vi "svfa_Check Waveform Parameter Continuity (1x1) [Dual FFT].vi"(0 "stimulus signal X [EUx]":waveform(dbl), 1 "restart averaging (F)":bool, 5 "response signal Y [EUy]":waveform(dbl), 7 "checks for channel parameter change":T1={"dt"=TRUE, "t0 continuity"=FALSE, "array length"=TRUE, "channel info"=TRUE, "name"=FALSE}, 11 "error in":errorcluster) -> (3 "dt":dbl, 4 "stimulus signal X [EUx]":waveform(dbl), 6 "response signal Y [EUy]":waveform(dbl), 8 "waveform parameter changed":bool, 14 "array length":i32, 15 "error out":errorcluster)   [LabVIEW 2017]
uses:
  <vilib>/addons/_NISVFA/_Shared subVIs/Common/svc_Check for Waveform Parameter Continuity (no state).vi
  <vilib>/addons/_NISVFA/_Shared subVIs/Common/svc_Get SV Channel Info.vi
  <vilib>/addons/_NISVFA/_Shared subVIs/Common/svc_Engineering Units to Unit Label.vi
  <vilib>/addons/_NISVFA/_Shared subVIs/Common/svc_Unit Label to Engineering Units.vi
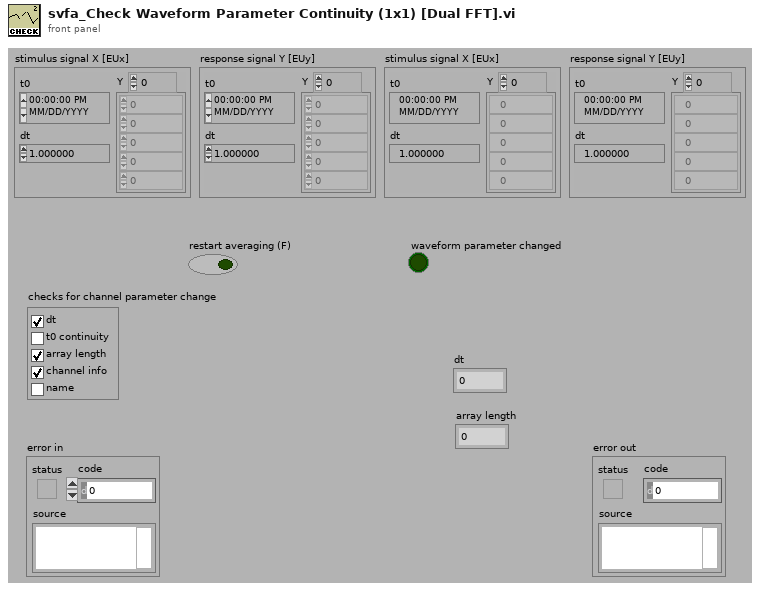
[diagram p1: front panel]
types:
  T1 = cluster{"dt":bool, "t0 continuity":bool, "array length":bool, "channel info":bool, "name":bool}
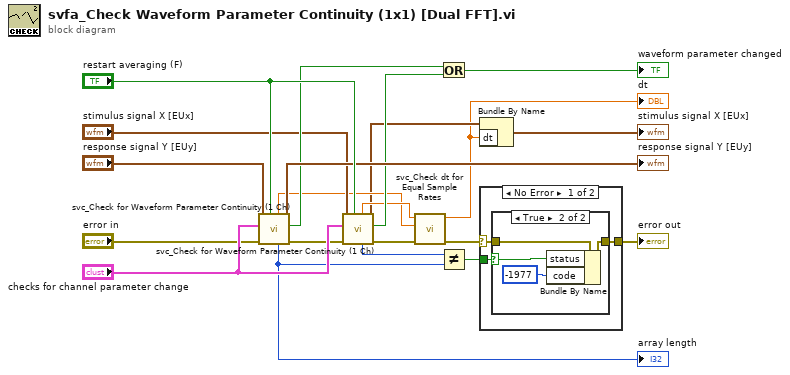
[diagram p0: block diagram]
diagram:
  n1 = call <vilib>:"svc_Check for Waveform Parameter Continuity (1 Ch).vi"("restart averaging (F)"="restart averaging (F)", "error in (no error)"="error in", "checks for channel parameter change"="checks for channel parameter change", "scaled signal [EU]"="response signal Y [EUy]") -> ("error out"=w19:errorcluster, "waveform parameter changed"=w14:bool, "dup scaled signal [EU]"=→"response signal Y [EUy]":waveform(dbl), "array length"=w8:i32, "dt"=w6:dbl)  [unwired: 2 in, 1 out]
  "array length" <- w8
  n2 = call <vilib>:"svc_Check for Waveform Parameter Continuity (1 Ch).vi"("restart averaging (F)"="restart averaging (F)", "error in (no error)"=w19, "checks for channel parameter change"="checks for channel parameter change", "scaled signal [EU]"="stimulus signal X [EUx]") -> ("error out"=w5:errorcluster, "waveform parameter changed"=w15:bool, "dup scaled signal [EU]"=w2:waveform(dbl), "array length"=w21:i32, "dt"=w7:dbl)  [unwired: 2 in, 1 out]
  n3 = call <vilib>:"svc_Check dt for Equal Sample Rates.vi"("error in (no error)"=w5, "dt Y"=w6, "dt X"=w7) -> ("error out"=w4:errorcluster, "dt Y"=w1:dbl)  [unwired: 7 in]
  "dt" <- w1
  n4 = Or(x=w14, y=w15) -> (x .or. y?=→"waveform parameter changed":bool)
  n5 = Not Equal?(x=w21, y=w8) -> (x != y?=w12:bool)
  n6 = Bundle By Name ("Build Waveform")(cluster=w2, "dt"=w1) -> (→"stimulus signal X [EUx]":waveform(dbl))
  n7 = case shown="No Error" w4 {
    selector: w4 -> [w23 w30]
    tunnel: w12 -> [w24 _]
    tunnel: [w22 w30] -> w9
    frame No Error {
      n8 = case shown="True" w24 {
        selector: w24 -> [_ w27]
        tunnel: [w25 w29] -> w22
        tunnel: w23 -> [w25 w26]
        frame False {
        }
        frame True {
          n9 = Bundle By Name(cluster=w26, "status"=w27, "code"=-1977) -> (w29:errorcluster)
        }
      }
    }
    frame Error {
    }
  }
  "error out" <- w9
